vi "SetTimeout.vi"(6 "Legacy?":bool, 8 "error in (no error)":errorcluster, 10 "Timeout (-1 = Don't timeout)":i32=-1) -> (0 "error out":errorcluster)   [LabVIEW 2011]
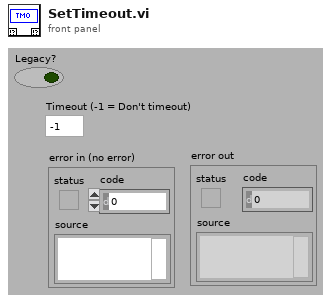
[diagram p1: front panel]
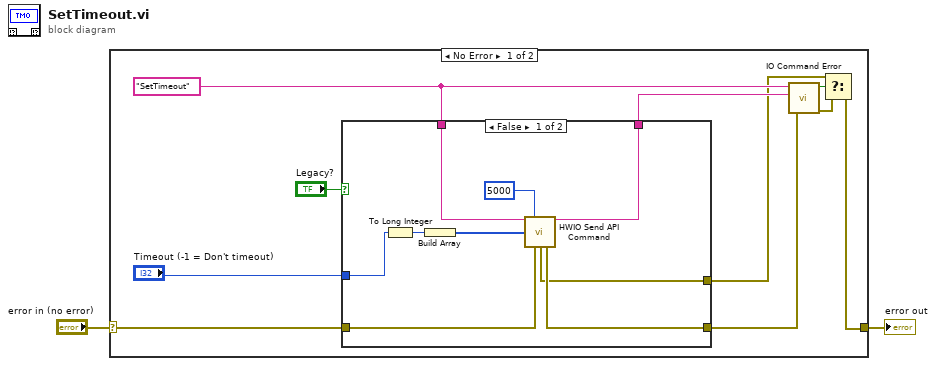
[diagram p0: block diagram]
diagram:
  n1 = case shown="No Error" "error in (no error)" {
    selector: "error in (no error)" -> [w8 w24]
    tunnel: [w4 w24] -> w2
    frame No Error {
      w10 = "SetTimeout"
      n2 = case shown="False" "Legacy?" {
        tunnel: "Timeout (-1 = Don't timeout)" -> [w21 _]
        tunnel: [w20 w23] -> w11
        tunnel: w10 -> [w19 w23]
        tunnel: [w18 w22] -> w9
        tunnel: w8 -> [w17 w22]
        tunnel: [w16 w22] -> w7
        frame False {
          n3 = To Long Integer(number=w21) -> (32bit integer=w14:i32)
          n4 = Build Array(w14) -> (w15:i32[])
          n5 = call "HWIO Send API Command.vi"("Action"=w19, "Timeout ms (5000)"=5000 ("PerCommand Timeout (ms)"), "Integer"=w15, "error in (no error)"=w17) -> ("Action out"=w20:string, "HWError"=w16:errorcluster, "error out"=w18:errorcluster)  [unwired: 4 in, 5 out]
        }
        frame True {
          # "No Timeout Feature for Legacy PIM api"
        }
      }
      n6 = call "IO Command Error.vi"("error in (no error)"=w9, "Command Returned (\"\")"=w11, "Command Sent (\"\")"=w10) -> ("error out"=w5:errorcluster, "HW ERR?"=w6:bool)  [unwired: 3 out]
      n7 = Select(t=w7, s=w6, f=w5) -> (s? t:f=w4:errorcluster)
    }
    frame Error {
    }
  }
  "error out" <- w2
